vi "unescape.vi"(11 "escaped string":string) -> (3 "unescaped":string)   [LabVIEW 2013, in "uniform resource locator.lvlib"]
uses:
  uniform resource locator.lvlib
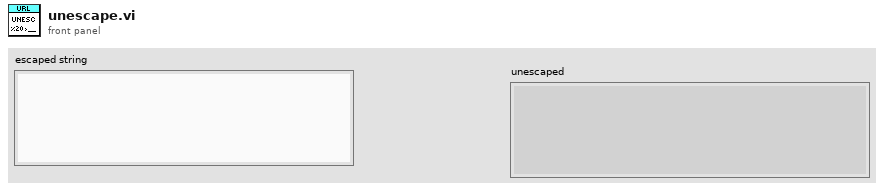
[diagram p1: front panel]
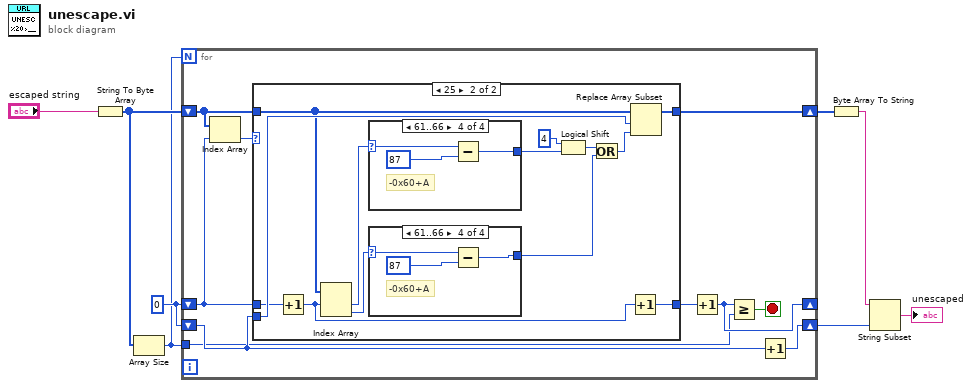
[diagram p0: block diagram]
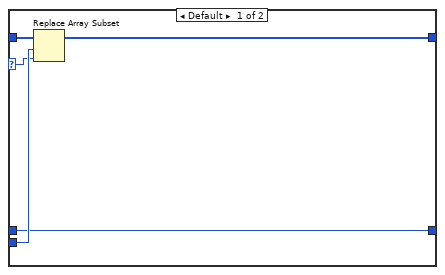
[diagram p2: hidden frame]
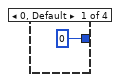
[diagram p3: hidden frame]
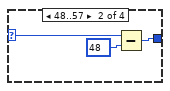
[diagram p4: hidden frame]
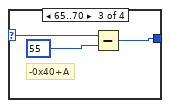
[diagram p5: hidden frame]
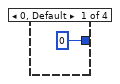
[diagram p6: hidden frame]
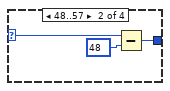
[diagram p7: hidden frame]
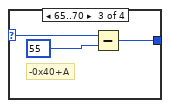
[diagram p8: hidden frame]
diagram:
  w7 = 0
  n1 = String To Byte Array(string="escaped string") -> (unsigned byte array=w2:u8[])
  n2 = Array Size(array=w2) -> (size(s)=w1:i32)
  n3 = for {
    N: w1 -> [_]
    shift-right: [w15] -> w6
    shift-left: w2 -> [w18]
    shift-right: [w10] -> _
    shift-left: w7 -> [w16]
    shift-right: [w14] -> w3
    shift-left: w7 -> [w12]
    tunnel: w1 -> [w9]
    stop <- w11 stop-if-true
    n4 = Index Array(array=w18, index=w16) -> (element=w17:u8)
    n5 = case shown="25" w17 {
      selector: w17 -> [w19 _]
      tunnel: w18 -> [w23 w33]
      tunnel: w16 -> [w20 w34]
      tunnel: [w22 w36] -> w15
      tunnel: w12 -> [w21 w35]
      tunnel: [w20 w31] -> w13
      frame Default {
        n6 = Replace Array Subset(array=w23, new element=w19, index=w21) -> (w22:u8[])
      }
      frame 37 {
        n7 = Increment(x=w34) -> (x+1=w32:i32)
        n8 = Index Array(array=w33, index #1=w32) -> (element #1=w30:u8, element #2=w29:u8)  [unwired: 1 in]
        n9 = case shown="61..66" w30 {
          selector: w30 -> [_ w50 w53 w56]
          tunnel: [u8 0 w48 w51 w54] -> w28
          frame 0, Default {
          }
          frame 48..57 {
            n10 = Subtract(x=w50, y=u8 48) -> (x-y=w48:u8)
          }
          frame 65..70 {
            # "-0x40+A"
            n11 = Subtract(x=w53, y=u8 55) -> (x-y=w51:u8)
          }
          frame 97..102 {
            # "-0x60+A"
            n12 = Subtract(x=w56, y=u8 87) -> (x-y=w54:u8)
          }
        }
        n13 = case shown="61..66" w29 {
          selector: w29 -> [_ w40 w43 w46]
          tunnel: [u8 0 w38 w41 w44] -> w26
          frame 0, Default {
          }
          frame 48..57 {
            n14 = Subtract(x=w40, y=u8 48) -> (x-y=w38:u8)
          }
          frame 65..70 {
            # "-0x40+A"
            n15 = Subtract(x=w43, y=u8 55) -> (x-y=w41:u8)
          }
          frame 97..102 {
            # "-0x60+A"
            n16 = Subtract(x=w46, y=u8 87) -> (x-y=w44:u8)
          }
        }
        n17 = Logical Shift(y=i16 4, x=w28) -> (x << y=w25:u8)
        n18 = Or(x=w25, y=w26) -> (x .or. y?=w24:u8)
        n19 = Increment(x=w32) -> (x+1=w31:i32)
        n20 = Replace Array Subset(array=w33, new element=w24, index=w35) -> (w36:u8[])
      }
    }
    n21 = Increment(x=w13) -> (x+1=w10:i32)
    n22 = Greater Or Equal?(x=w10, y=w9) -> (x >= y?=w11:bool)
    n23 = Increment(x=w12) -> (x+1=w14:i32)
  }
  n24 = Byte Array To String(unsigned byte array=w6) -> (string=w5:string)
  n25 = String Subset(string=w5, length (rest)=w3) -> (substring=→"unescaped":string)  [unwired: 1 in]
